vi "Waveform Lookup.vi"(9 "nelem":u16, 10 "table":refnum<k21>, 11 "accumulator":u32) -> (3 "value":i16)   [LabVIEW 2017, in "Analog IO.lvlib" / "Analog Output.lvclass"]
uses:
  Analog Output.lvclass
  <vilib>/rvi/DataTransferAndStorage/Container/Common/niFpgaContainerExecOnDevCompGetState.vi
  <vilib>/rvi/Emulation/niFpgaEmulationIsFPGAContextNoSignature.vi
  <vilib>/rvi/DataTransferAndStorage/Container/Common/niFpgaContainerGetUniqueNameForEmu.vi
  <vilib>/rvi/Emulation/niFpgaProcessEmulError.vi
  <vilib>/rvi/Emulation/niFpgaSctlEmulationGetInTimedLoop.vi
  <vilib>/rvi/errors/nirviReportUnexpectedCaseInternalError (U32).vi
  <vilib>/rvi/Memory/Memory_Emulation/niFpgaMemoryEmulationCacheClearOnFirstRun.vi
  <vilib>/rvi/Memory/Memory_Emulation/nirvimemoryEmulationManagerCache_MakeExclusive.vi
  <vilib>/rvi/Memory/Memory_Emulation/niFpgaMemoryEmulationValidateCache.vi
  <vilib>/rvi/Memory/Memory_Emulation/nirvimemoryEmulationManagerCache_InsertValue.vi
  <vilib>/Utility/error.llb/Clear Errors.vi
  <vilib>/rvi/Memory/Memory_Emulation/nirvimemoryEmulationManagerCache_ReleaseExclusive.vi
  <vilib>/rvi/Memory/Memory_Emulation/nirvimemoryEmulationManagerCache_GetValue.vi
  <vilib>/rvi/Memory/Memory_Emulation/nirvimemoryEmulationManagerCache_SetValue.vi
  <vilib>/rvi/Emulation/niFpgaSctlEmulationResourceMgr.vi
  <vilib>/rvi/DataTransferAndStorage/Container/XNode/niFpgaContainer.xnode
  <vilib>/rvi/Memory/Memory_Emulation/niFpgaMemoryEmulationRefIn.vi
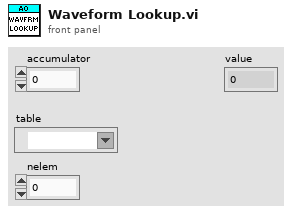
[diagram p1: front panel]
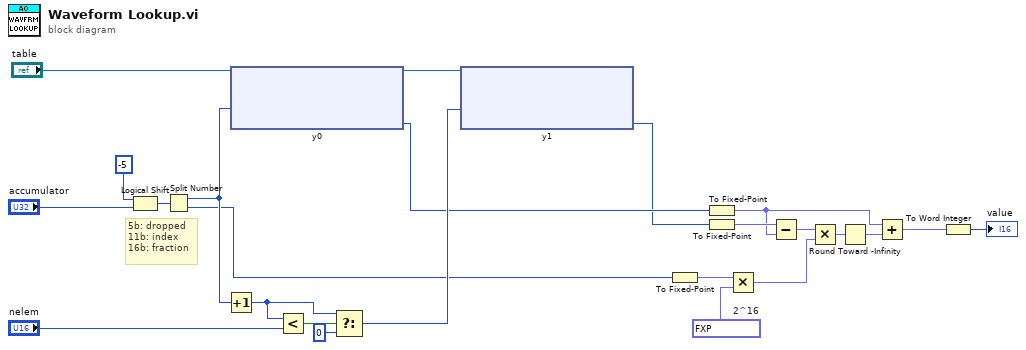
[diagram p0: block diagram]
diagram:
  w5 = fxp<+/-,16,0> 1.52587890625e-05  # 2^16
  # "5b: dropped\n11b: index\n16b: fraction"
  n1 = Logical Shift(y=i16 -5, x="accumulator") -> (x << y=w23:u32)
  n2 = Split Number(x=w23) -> (hi(x)=w16:u16, lo(x)=w4:u16)
  n3 = Increment(x=w16) -> (x+1=w20:u16)
  n4 = xnode "y0"("Address"=w16, "Memory In"="table") -> ("Data"=w14:i16, "Memory Out"=w17:refnum<k21>)
  n5 = Less?(x=w20, y="nelem") -> (x < y?=w21:bool)
  n6 = Select(t=w20, s=w21, f=u16 0) -> (s? t:f=w15:u16)
  n7 = xnode "y1"("Address"=w15, "Memory In"=w17) -> ("Data"=w13:i16)  [unwired: 1 out]
  n8 = To Fixed-Point(number=w4) -> (fixed-point=w1:fxp<+,16,16>)  [unwired: 1 in]
  n9 = To Fixed-Point(number=w14) -> (fixed-point=w8:fxp<+/-,16,16>)  [unwired: 1 in]
  n10 = To Fixed-Point(number=w13) -> (fixed-point=w12:fxp<+/-,16,16>)  [unwired: 1 in]
  n11 = Multiply(x=w1, y=w5) -> (x*y=w7:fxp<+/-,32,16>)
  n12 = Subtract(x=w12, y=w8) -> (x-y=w11:fxp<+/-,17,17>)
  n13 = Multiply(x=w11, y=w7) -> (x*y=w10:fxp<+/-,48,32>)
  n14 = Round Toward -Infinity(1:w10) -> (0:w9:fxp<+/-,32,32>)
  n15 = Add(x=w8, y=w9) -> (x+y=w3:fxp<+/-,16,16>)
  n16 = To Word Integer(number=w3) -> (16bit integer=→"value":i16)
